vi "CSV_AppendNewColumns.vi"(8 "error in (no error)":errorcluster, 10 "New/Existing CSV file path":path, 11 "LabVIEW Data":variant) -> (0 "error out":errorcluster)   [LabVIEW 2015, in "LVdataToTableData.lvlib"]
uses:
  LVdataToTableData.lvlib
  <userlib>/_OpenG.lib/file/file.llb/File Exists - Scalar__ogtk.vi
  <vilib>/Utility/file.llb/Write Delimited Spreadsheet (string).vi
  <vilib>/Utility/file.llb/Read Delimited Spreadsheet (string).vi
panel:
  # "Connector Pane"
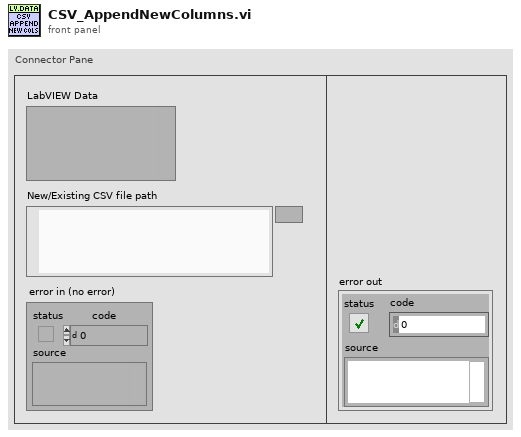
[diagram p1: front panel]
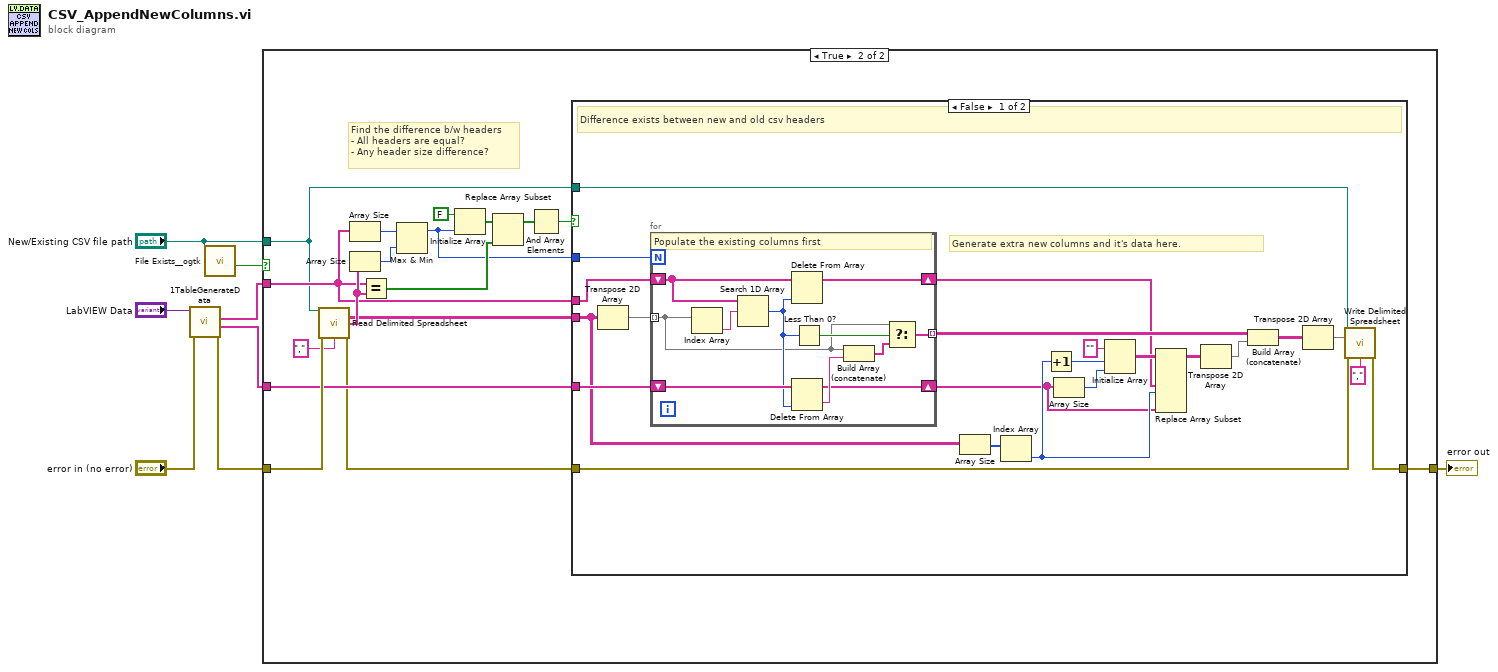
[diagram p0: block diagram]
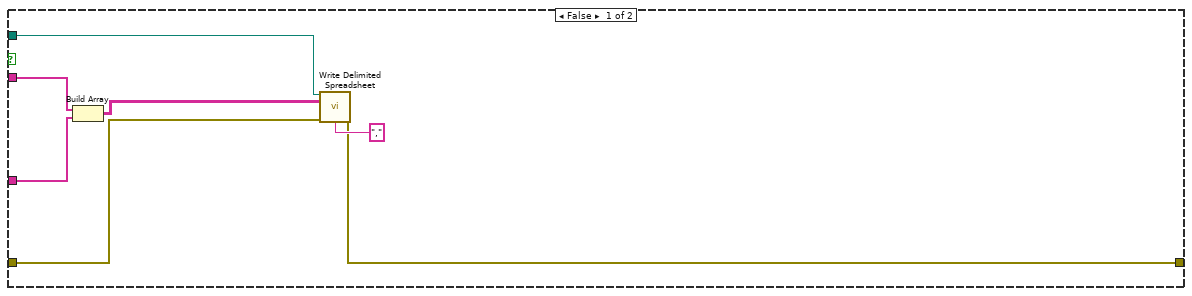
[diagram p2: hidden frame]
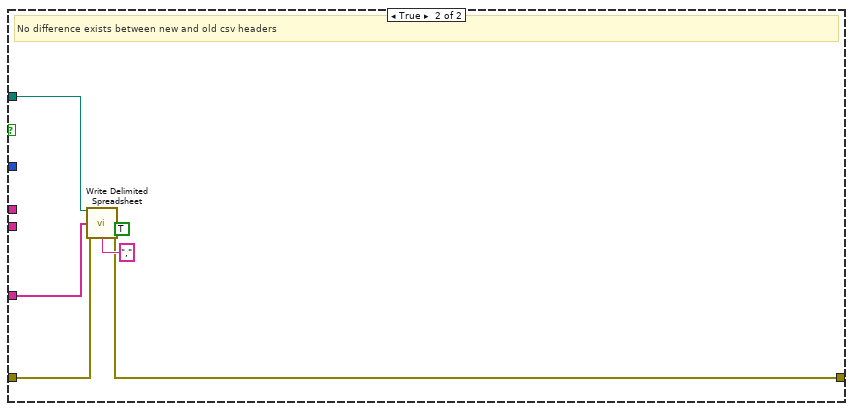
[diagram p3: hidden frame]
diagram:
  n1 = call "1TableGenerateData.vi"("error in (no error)"="error in (no error)", "Cluster Variant"="LabVIEW Data") -> ("error out"=w7:errorcluster, "Data"=w6:string[], "Headers"=w5:string[])  [unwired: 5 in, 2 out]
  n2 = call-poly <userlib>:"File Exists__ogtk.vi"("file path"="New/Existing CSV file path") -> ("exists"=w2:bool)  [unwired: 6 in, 1 out]
  n3 = case shown="True" w2 {
    tunnel: w7 -> [w10 w32]
    tunnel: w6 -> [w13 w31]
    tunnel: w5 -> [w14 w22]
    tunnel: "New/Existing CSV file path" -> [w11 w19]
    tunnel: [w9 w16] -> w1
    frame False {
      n4 = Build Array(w14, w13) -> (w12:string[][])
      n5 = call-poly <vilib>:"Write Delimited Spreadsheet.vi"("file path (dialog if empty)"=w11, "2D data"=w12, "error in (no error)"=w10, "delimiter (\\t)"="," ("delimiter (\\t)")) -> ("error out"=w9:errorcluster)  [unwired: 10 in, 1 out]
    }
    frame True {
      # "Find the difference b/w headers\n- All headers are equal?\n- Any header size difference?"
      n6 = call-poly <vilib>:"Read Delimited Spreadsheet.vi"("file path (dialog if empty)"=w19, "error in (no error)"=w32, "delimiter (\\t)"="," ("delimiter (\\t)")) -> ("all rows"=w21:string[][], "first row"=w30:string[], "error out"=w20:errorcluster)  [unwired: 7 in, 3 out]
      n7 = Array Size(array=w22) -> (size(s)=w27:i32)
      n8 = Array Size(array=w30) -> (size(s)=w28:i32)
      n9 = Equal?(x=w22, y=w30) -> (x = y?=w25:bool[])
      n10 = Max & Min(x=w27, y=w28) -> (max(x,y)=w23:i32)  [unwired: 1 out]
      n11 = Initialize Array(FALSE, w23) -> (w26:bool[])
      n12 = Replace Array Subset(array=w26, new element=w25) -> (w24:bool[])  [unwired: 1 in]
      n13 = And Array Elements(Boolean array=w24) -> (logical AND=w18:bool)
      n14 = case shown="False" w18 {
        tunnel: w31 -> [w54 w70]
        tunnel: w23 -> [w53 _]
        tunnel: w22 -> [w48 _]
        tunnel: w21 -> [w47 _]
        tunnel: w20 -> [w52 w67]
        tunnel: w19 -> [w51 w71]
        tunnel: [w33 w66] -> w16
        frame False {
          # "Generate extra new columns and it's data here."
          # "Difference exists between new and old csv headers"
          n15 = Transpose 2D Array(2D array=w47) -> (transposed array=w34:string[][])
          n16 = for {
            N: w53 -> [_]
            tunnel: w34 -> [w55] mode=indexing
            tunnel: [w56] -> w50 mode=indexing
            shift-right: [w61] -> w42
            shift-left: w48 -> [w62]
            shift-right: [w60] -> w40
            shift-left: w54 -> [w65]
            # "Populate the existing columns first"
            n17 = Index Array(array=w55) -> (element=w63:string)  [unwired: 1 in]
            n18 = Search 1D Array(1D array=w62, element=w63) -> (index of element=w59:i32)  [unwired: 1 in]
            n19 = Delete From Array(array=w62, index=w59) -> (array with subset deleted=w61:string[])  [unwired: 1 in, 1 out]
            n20 = Delete From Array(array=w65, index=w59) -> (deleted portion=w64:string, array with subset deleted=w60:string[])  [unwired: 1 in]
            n21 = Less Than 0?(x=w59) -> (x < 0?=w58:bool)
            n22 = Build Array (concatenate)(w55, w64) -> (w57:string[])
            n23 = Select(t=w55, s=w58, f=w57) -> (s? t:f=w56:string[])
          }
          n24 = Array Size(array=w47) -> (size(s)=w46:i32[])
          n25 = Index Array(array=w46) -> (element=w41:i32)  [unwired: 1 in]
          n26 = Increment(x=w41) -> (x+1=w35:i32)
          n27 = Array Size(array=w40) -> (size(s)=w44:i32)
          n28 = Initialize Array("", w35, w44) -> (w43:string[][])
          n29 = Replace Array Subset(array=w43, new element #1=w42, new element #2=w40, index (row) #2=w41) -> (w38:string[][])  [unwired: 3 in]
          n30 = Transpose 2D Array(2D array=w38) -> (transposed array=w37:string[][])
          n31 = Build Array (concatenate)(w50, w37) -> (w39:string[][])
          n32 = Transpose 2D Array(2D array=w39) -> (transposed array=w36:string[][])
          n33 = call-poly <vilib>:"Write Delimited Spreadsheet.vi"("file path (dialog if empty)"=w51, "2D data"=w36, "error in (no error)"=w52, "delimiter (\\t)"="," ("delimiter (\\t)")) -> ("error out"=w33:errorcluster)  [unwired: 10 in, 1 out]
        }
        frame True {
          # "No difference exists between new and old csv headers"
          n34 = call-poly <vilib>:"Write Delimited Spreadsheet.vi"("file path (dialog if empty)"=w71, "1D data"=w70, "append to file? (F)"=TRUE, "error in (no error)"=w67, "delimiter (\\t)"="," ("delimiter (\\t)")) -> ("error out"=w66:errorcluster)  [unwired: 9 in, 1 out]
        }
      }
    }
  }
  "error out" <- w1
